vi "repeat cycle_exponential up.vi"(8 "error in (no error)":errorcluster caption="에러 입력(에러 없음)", 10 "waveform in":waveform(dbl), 11 "Waveform Obj 입력":refnum<class "PWL_DW7802.lvclass">) -> (0 "error out":errorcluster caption="에러 출력", 2 "waveform out":waveform(dbl), 3 "Waveform Obj 출력":refnum<class "PWL_DW7802.lvclass">)   [LabVIEW 2020, in "PWL_DW7802.lvclass"]
uses:
  PWL_DW7802.lvclass
  Waveform Gen/Waveform Gen.lvclass/Waveform Gen.ctl
  PWL/PWL.lvclass/PWL.ctl
  Waveform Gen/Accessors/Read cycle.vi
  Waveform Gen/Accessors/Read scale.vi
  PWL/Accessors/Read previous pwl scale.vi
  <vilib>/Waveform/WDTOps.llb/WDT Number of Waveform Samples DBL.vi
  <vilib>/Waveform/WDTOps.llb/WDT Get Waveform Subset DBL.vi
  <vilib>/Waveform/WDTOps.llb/WDT Append Waveforms DBL.vi
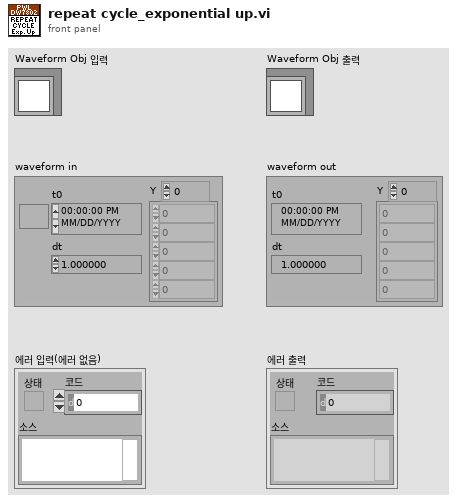
[diagram p1: front panel]
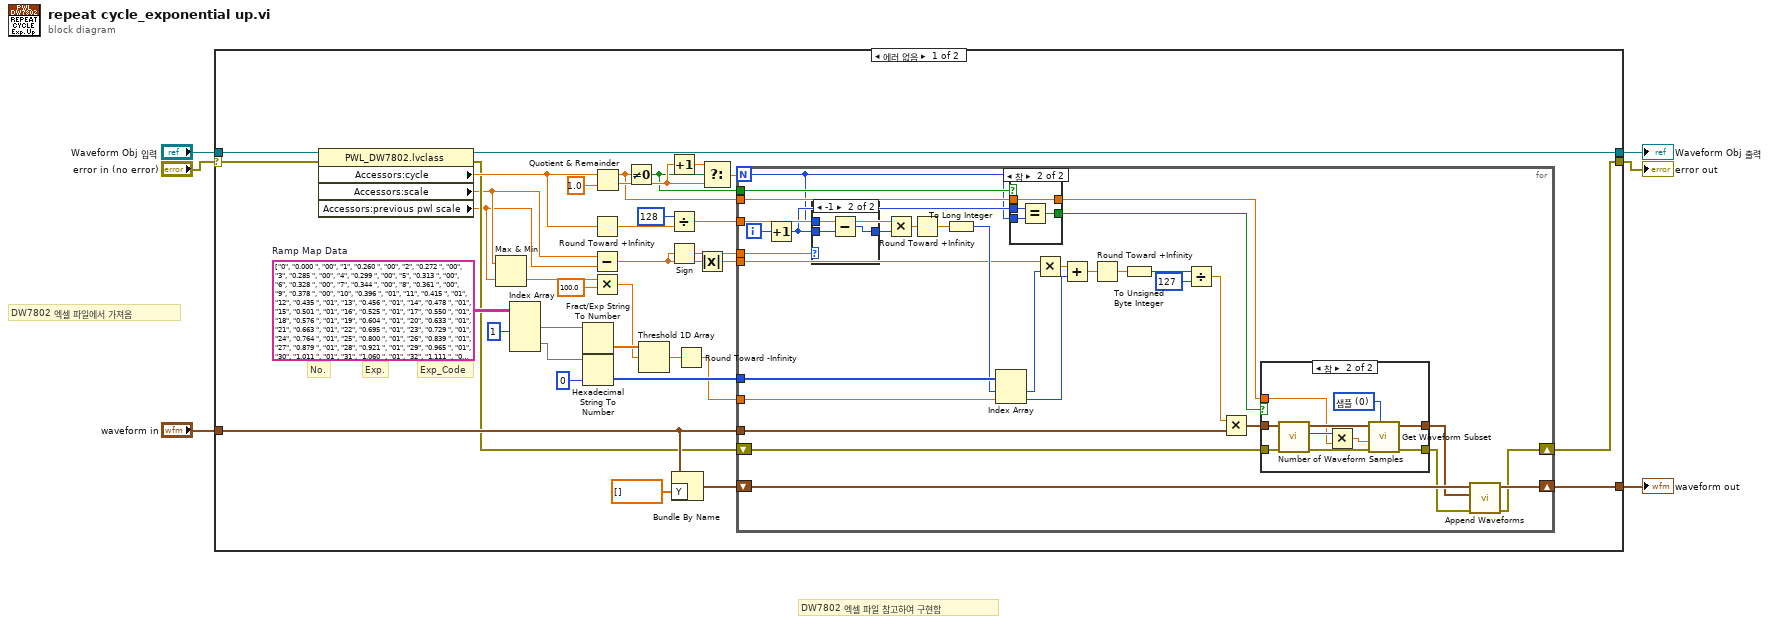
[diagram p0: block diagram]
diagram:
  # "DW7802 엑셀 파일에서 가져옴"
  # "DW7802 엑셀 파일 참고하여 구현함"
  n1 = case shown="에러 없음" "error in (no error)" {
    selector: "error in (no error)" -> [w41 w95]
    tunnel: "Waveform Obj 입력" -> [w42 w96]
    tunnel: [w40 w96] -> w4
    tunnel: [w19 w95] -> w3
    tunnel: "waveform in" -> [w26 _]
    tunnel: [w18 _] -> w1
    frame No Error {
      w34 = string[][] [["0", "0.000 ", "00"], ["1", "0.260 ", "00"], ["2", "0.272 ", "00"], ["3", "0.285 ", "00"], ["4", "0.299 ", "00"], ["5", "0.313 ", "00"], ["6", "0.328 ", "00"], ["7", "0.344 ", "00"], ["8", "0.361 ", "00"], ["9", "0.378 ", "00"], ["10", "0.396 ", "01"], ["11", "0.415 ", "01"], ["12", "0.435 ", "01"], ["13", "0.456 ", "01"], ["14", "0.478 ", "01"], ["15", "0.501 ", "01"], ["16", "0.525 ", "01"], ["17", "0.550 ", "01"], ["18", "0.576 ", "01"], ["19", "0.604 ", "01"], ["20", "0.633 ", "01"], ["21", "0.663 ", "01"], ["22", "0.695 ", "01"], ["23", "0.729 ", "01"], ["24", "0.764 ", "01"], ["25", "0.800 ", "01"], ["26", "0.839 ", "01"], ["27", "0.879 ", "01"], ["28", "0.921 ", "01"], ["29", "0.965 ", "01"], ["30", "1.011 ", "01"], ["31", "1.060 ", "01"], ["32", "1.111 ", "01"], ["33", "1.164 ", "01"], ["34", "1.220 ", "02"], ["35", "1.279 ", "02"], ["36", "1.340 ", "02"], ["37", "1.404 ", "02"], ["38", "1.472 ", "02"], ["39", "1.542 ", "02"], ["40", "1.616 ", "02"], ["41", "1.694 ", "02"], ["42", "1.775 ", "02"], ["43", "1.860 ", "02"], ["44", "1.950 ", "02"], ["45", "2.043 ", "03"], ["46", "2.141 ", "03"], ["47", "2.244 ", "03"], ["48", "2.352 ", "03"], ["49", "2.465 ", "03"], ["50", "2.583 ", "03"], ["51", "2.707 ", "03"], ["52", "2.837 ", "04"], ["53", "2.973 ", "04"], ["54", "3.116 ", "04"], ["55", "3.265 ", "04"], ["56", "3.422 ", "04"], ["57", "3.586 ", "05"], ["58", "3.758 ", "05"], ["59", "3.938 ", "05"], ["60", "4.127 ", "05"], ["61", "4.326 ", "05"], ["62", "4.533 ", "06"], ["63", "4.751 ", "06"], ["64", "4.979 ", "06"], ["65", "5.218 ", "07"], ["66", "5.468 ", "07"], ["67", "5.730 ", "07"], ["68", "6.005 ", "08"], ["69", "6.294 ", "08"], ["70", "6.596 ", "08"], ["71", "6.912 ", "09"], ["72", "7.244 ", "09"], ["73", "7.592 ", "0A"], ["74", "7.956 ", "0A"], ["75", "8.338 ", "0B"], ["76", "8.738 ", "0B"], ["77", "9.157 ", "0C"], ["78", "9.597 ", "0C"], ["79", "10.057 ", "0D"], ["80", "10.540 ", "0D"], ["81", "11.046 ", "0E"], ["82", "11.576 ", "0F"], ["83", "12.131 ", "0F"], ["84", "12.714 ", "10"], ["85", "13.324 ", "11"], ["86", "13.963 ", "12"], ["87", "14.633 ", "13"], ["88", "15.335 ", "13"], ["89", "16.071 ", "14"], ["90", "16.843 ", "15"], ["91", "17.651 ", "16"], ["92", "18.498 ", "17"], ["93", "19.386 ", "19"], ["94", "20.316 ", "1A"], ["95", "21.291 ", "1B"], ["96", "22.313 ", "1C"], ["97", "23.384 ", "1E"], ["98", "24.506 ", "1F"], ["99", "25.682 ", "21"], ["100", "26.915 ", "22"], ["101", "28.206 ", "24"], ["102", "29.560 ", "26"], ["103", "30.979 ", "27"], ["104", "32.465 ", "29"], ["105", "34.023 ", "2B"], ["106", "35.656 ", "2D"], ["107", "37.367 ", "2F"], ["108", "39.161 ", "32"], ["109", "41.040 ", "34"], ["110", "43.009 ", "37"], ["111", "45.074 ", "39"], ["112", "47.237 ", "3C"], ["113", "49.504 ", "3F"], ["114", "51.879 ", "42"], ["115", "54.369 ", "45"], ["116", "56.978 ", "48"], ["117", "59.713 ", "4C"], ["118", "62.578 ", "4F"], ["119", "65.582 ", "53"], ["120", "68.729 ", "57"], ["121", "72.027 ", "5B"], ["122", "75.484 ", "60"], ["123", "79.107 ", "64"], ["124", "82.903 ", "69"], ["125", "86.882 ", "6E"], ["126", "91.051 ", "74"], ["127", "95.421 ", "79"], ["128", "100.000 ", "7F"]]  # Ramp Map Data
      # "Exp_Code"
      # "Exp."
      # "No."
      n2 = property class="PWL_DW7802.lvclass"(reference=w42, error in=w41) -> (reference out=w40:refnum<class "PWL_DW7802.lvclass">, error out=w20:errorcluster, "Accessors:cycle"=w30:dbl, "Accessors:scale"=w9:dbl, "Accessors:previous pwl scale"=w8:dbl)
      n3 = Max & Min(x=w9, y=w8) -> (min(x,y)=w7:dbl)  [unwired: 1 out]
      n4 = Index Array(array=w34, index (col) #1=1 ("비활성화된 인덱스 (열)")) -> (element #1=w39:string[], element #2=w32:string[])  [unwired: 3 in]
      n5 = Fract/Exp String To Number(string=w39) -> (number=w15:dbl[])  [unwired: 3 in, 1 out]
      n6 = Hexadecimal String To Number(string=w32, default (0uL)=u8 0) -> (number=w38:u8[])  [unwired: 1 in, 1 out]
      n7 = Round Toward +Infinity(x=w30) -> (ceil(x): smallest int >= x=w17:dbl)
      n8 = Subtract(x=w9, y=w8) -> (x-y=w12:dbl)
      n9 = Multiply(x=w7, y=100.0) -> (x*y=w13:dbl)
      n10 = Quotient & Remainder(x=w30, y=1.0) -> (x-y*floor(x/y)=w21:dbl, floor(x/y)=w23:dbl)
      n11 = Not Equal To 0?(x=w21) -> (x != 0?=w22:bool)
      n12 = Threshold 1D Array(2:w13, 3:w15) -> (0:w16:dbl)  [unwired: 1 in]
      n13 = Increment(x=w23) -> (x+1=w28:dbl)
      n14 = Divide(x=u8 128 ("y"), y=w17) -> (x/y=w37:dbl)
      n15 = Sign(1:w12) -> (0:w11:dbl)
      n16 = Bundle By Name(cluster=w26, "Y"=dbl[] []) -> (w24:waveform(dbl))
      n17 = Round Toward -Infinity(1:w16) -> (0:w14:dbl)
      n18 = Absolute Value(x=w12) -> (abs(x)=w10:dbl)
      n19 = Select(t=w28, s=w22, f=w23) -> (s? t:f=w27:dbl)
      n20 = for {
        N: w27 -> [w43]
        tunnel: w37 -> [w74]
        tunnel: w38 -> [w73]
        tunnel: w10 -> [w68]
        tunnel: w26 -> [w60]
        shift-right: [w52] -> w18
        shift-left: w24 -> [w61]
        tunnel: w22 -> [w58]
        tunnel: w21 -> [w57]
        shift-right: [w49] -> w19
        shift-left: w20 -> [w51]
        tunnel: w14 -> [w48]
        tunnel: w11 -> [w47]
        i -> [w46]
        n21 = Increment(x=w46) -> (x+1=w45:i32)
        n22 = case shown="-1" w47 {
          tunnel: w45 -> [w75 w76]
          tunnel: [w75 w77] -> w44
          tunnel: w43 -> [_ w78]
          frame 0, Default {
          }
          frame -1 {
            n23 = Subtract(x=w78, y=w76) -> (x-y=w77:i32)
          }
        }
        n24 = Multiply(x=w74, y=w44) -> (x*y=w72:dbl)
        n25 = Round Toward +Infinity(x=w72) -> (ceil(x): smallest int >= x=w71:dbl)
        n26 = To Long Integer(number=w71) -> (32bit integer=w70:i32)
        n27 = Index Array(array=w73, index #1=w70, index #2=w48) -> (element #1=w69:u8, element #2=w66:u8)
        n28 = case shown="참" w58 {
          tunnel: w57 -> [_ w92]
          tunnel: w45 -> [_ w94]
          tunnel: w43 -> [_ w93]
          tunnel: [_ w92] -> w55
          tunnel: [_ w91] -> w56
          frame False {
          }
          frame True {
            n29 = Equal?(x=w94, y=w93) -> (x = y?=w91:bool)
          }
        }
        n30 = Multiply(x=w68, y=w69) -> (x*y=w67:dbl)
        n31 = Add(x=w67, y=w66) -> (x+y=w65:dbl)
        n32 = Round Toward +Infinity(x=w65) -> (ceil(x): smallest int >= x=w64:dbl)
        n33 = To Unsigned Byte Integer(number=w64) -> (unsigned 8bit integer=w63:u8)
        n34 = Divide(x=w63, y=u8 127) -> (x/y=w59:dbl)
        n35 = Multiply(x=w59, y=w60) -> (x*y=w54:waveform(dbl))
        n36 = case shown="참" w56 {
          tunnel: w55 -> [_ w84]
          tunnel: w54 -> [w80 w85]
          tunnel: [w80 w83] -> w53
          tunnel: w51 -> [w79 w82]
          tunnel: [w79 w81] -> w50
          frame False {
          }
          frame True {
            w86 = u16 0 items=["샘플", "상대 시간"] ("start/duration format")
            n37 = call-poly <vilib>:"Number of Waveform Samples.vi"("error in (no error)"=w82, "waveform in"=w85) -> ("error out"=w89:errorcluster, "number of samples"=w87:i32, "waveform out"=w90:waveform(dbl))  [unwired: 7 in]
            n38 = Multiply(x=w87, y=w84) -> (x*y=w88:dbl)
            n39 = call-poly <vilib>:"Get Waveform Subset.vi"("start/duration format"=w86, "error in (no error)"=w89, "duration"=w88, "waveform in"=w90) -> ("error out"=w81:errorcluster, "waveform out"=w83:waveform(dbl))  [unwired: 2 in, 2 out]
          }
        }
        n40 = call-poly <vilib>:"Append Waveforms.vi"("error in (no error)"=w50, "waveform B"=w53, "waveform A"=w61) -> ("error out"=w49:errorcluster, "waveform out"=w52:waveform(dbl))  [unwired: 7 in]
      }
    }
    frame Error {
    }
  }
  "error out" <- w3
  "Waveform Obj 출력" <- w4
  "waveform out" <- w1
